vi "GlobalGetInitialisationStatus.vi"() -> ()   [LabVIEW 2013]
panel:
  out "DeviceStartUpDone":bool
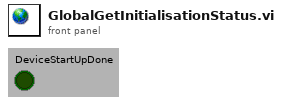
[diagram p1: front panel]
diagram:
